vi "niDTS WLAN INSTR TX Configure.vi"(6 "Port Names":string[](array[string])=["RF0/Port0", "RF1/Port1", "RF0/Port6", "RF1/Port7"], 8 "error in (no error)":errorcluster, 9 "Payload length bytes":i32, 10 "Channel Secondary Factor":enum16{"-1", "1", "0"}(ring)=enum."1", 11 "niDTS WLAN INSTR TX in":refnum<class "niDTS WLAN INSTR TX.lvclass">) -> (0 "error out":errorcluster, 3 "niDTS WLAN INSTR TX out":refnum<class "niDTS WLAN INSTR TX.lvclass">)   [LabVIEW 2015, in "niDTS WLAN.lvlib" / "niDTS WLAN INSTR TX.lvclass"]
uses:
  niDTS WLAN INSTR TX.lvclass
  niDTS WLAN INSTR TX.lvclass/niDTS WLAN INSTR TX.ctl
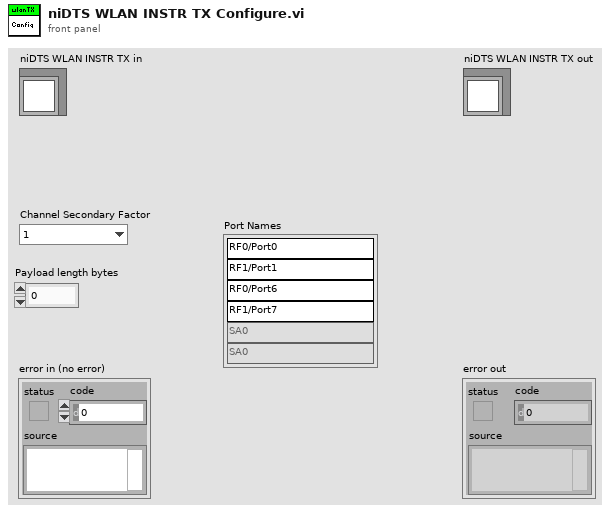
[diagram p1: front panel]
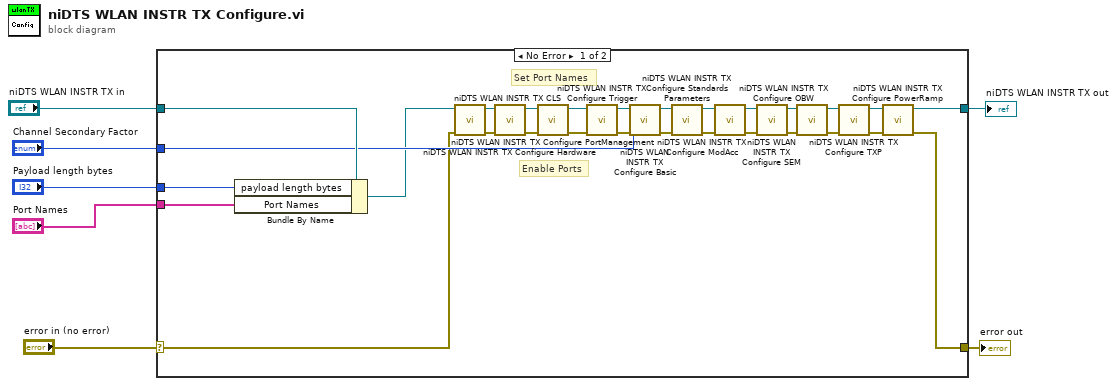
[diagram p0: block diagram]
diagram:
  n1 = case shown="No Error" "error in (no error)" {
    selector: "error in (no error)" -> [w9 w37]
    tunnel: [w12 w37] -> w6
    tunnel: [w14 w36] -> w4
    tunnel: "niDTS WLAN INSTR TX in" -> [w35 w36]
    tunnel: "Channel Secondary Factor" -> [w25 _]
    tunnel: "Payload length bytes" -> [w33 _]
    tunnel: "Port Names" -> [w16 _]
    frame No Error {
      # "Set Port Names"
      # "Enable Ports"
      n2 = Bundle By Name(cluster=w35, "payload length bytes"=w33, "Port Names"=w16) -> (w8:refnum<class "niDTS WLAN INSTR TX.lvclass">)
      n3 = call-dynamic "niDTS WLAN INSTR TX CLS.vi"("error in (no error)"=w9, "niDTS WLAN INSTR TX in"=w8) -> ("error out"=w10:errorcluster, "niDTS WLAN INSTR TX out"=w11:refnum<class "niDTS WLAN INSTR TX.lvclass">)  [unwired: 8 in]
      n4 = call-dynamic "niDTS WLAN INSTR TX Configure Hardware.vi"("error in (no error)"=w10, "niDTS WLAN INSTR TX in"=w11) -> ("error out"=w23:errorcluster, "niDTS WLAN INSTR TX out"=w24:refnum<class "niDTS WLAN INSTR TX.lvclass">)  [unwired: 8 in]
      n5 = call-dynamic "niDTS WLAN INSTR TX Configure PortManagement.vi"("error in (no error)"=w23, "niDTS WLAN INSTR TX in"=w24) -> ("error out"=w21:errorcluster, "niDTS WLAN INSTR TX out"=w22:refnum<class "niDTS WLAN INSTR TX.lvclass">)  [unwired: 8 in]
      n6 = call "niDTS WLAN INSTR TX Configure Trigger.vi"("error in (no error)"=w21, "niDTS WLAN INSTR TX in"=w22) -> ("error out"=w19:errorcluster, "niDTS WLAN INSTR TX out"=w20:refnum<class "niDTS WLAN INSTR TX.lvclass">)  [unwired: 8 in]
      n7 = call-dynamic "niDTS WLAN INSTR TX Configure Basic.vi"("error in (no error)"=w19, "Channel Secondary Factor"=w25, "niDTS WLAN INSTR TX in"=w20) -> ("error out"=w17:errorcluster, "niDTS WLAN INSTR TX out"=w18:refnum<class "niDTS WLAN INSTR TX.lvclass">)  [unwired: 7 in]
      n8 = call-dynamic "niDTS WLAN INSTR TX Configure Standards Parameters.vi"("error in (no error)"=w17, "niDTS WLAN INSTR TX in"=w18) -> ("error out"=w31:errorcluster, "niDTS WLAN INSTR TX out"=w34:refnum<class "niDTS WLAN INSTR TX.lvclass">)  [unwired: 8 in]
      n9 = call-dynamic "niDTS WLAN INSTR TX Configure ModAcc.vi"("error in (no error)"=w31, "niDTS WLAN INSTR TX in"=w34) -> ("error out"=w29:errorcluster, "niDTS WLAN INSTR TX out"=w32:refnum<class "niDTS WLAN INSTR TX.lvclass">)  [unwired: 8 in]
      n10 = call-dynamic "niDTS WLAN INSTR TX Configure SEM.vi"("error in (no error)"=w29, "niDTS WLAN INSTR TX in"=w32) -> ("error out"=w27:errorcluster, "niDTS WLAN INSTR TX out"=w30:refnum<class "niDTS WLAN INSTR TX.lvclass">)  [unwired: 8 in]
      n11 = call-dynamic "niDTS WLAN INSTR TX Configure OBW.vi"("error in (no error)"=w27, "niDTS WLAN INSTR TX in"=w30) -> ("error out"=w26:errorcluster, "niDTS WLAN INSTR TX out"=w28:refnum<class "niDTS WLAN INSTR TX.lvclass">)  [unwired: 8 in]
      n12 = call-dynamic "niDTS WLAN INSTR TX Configure TXP.vi"("error in (no error)"=w26, "niDTS WLAN INSTR TX in"=w28) -> ("error out"=w13:errorcluster, "niDTS WLAN INSTR TX out"=w15:refnum<class "niDTS WLAN INSTR TX.lvclass">)  [unwired: 8 in]
      n13 = call-dynamic "niDTS WLAN INSTR TX Configure PowerRamp.vi"("error in (no error)"=w13, "niDTS WLAN INSTR TX in"=w15) -> ("error out"=w12:errorcluster, "niDTS WLAN INSTR TX out"=w14:refnum<class "niDTS WLAN INSTR TX.lvclass">)  [unwired: 8 in]
    }
    frame Error {
    }
  }
  "error out" <- w6
  "niDTS WLAN INSTR TX out" <- w4
